vi "Initialize Attributes.vi"(8 "error in (no error)":errorcluster, 10 "Attribute Data":variant, 11 "CS++DIM-Client in":refnum<class "CS++DIM-Client.lvclass">) -> (0 "error out":errorcluster, 2 "Found?":bool, 3 "CS++DIM-Client out":refnum<class "CS++DIM-Client.lvclass">)   [LabVIEW 2016, in "CS++DIM-Client.lvlib" / "CS++DIM-Client.lvclass"]
doc: "Initialize object attribute.\n\nUnique resources should be allocated elsewhere!"
uses:
  CS++DIM-Client.lvclass
  CS++DIM-Client.lvclass/CS++DIM-Client.ctl
  CSPP_Core/Actors/CS++GUIActor/CS++GUIActor.lvclass
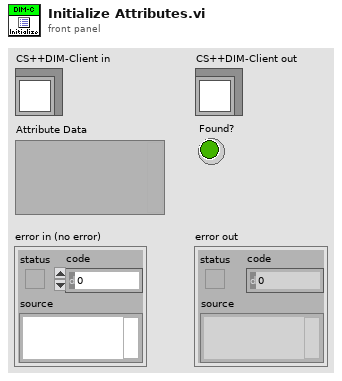
[diagram p1: front panel]
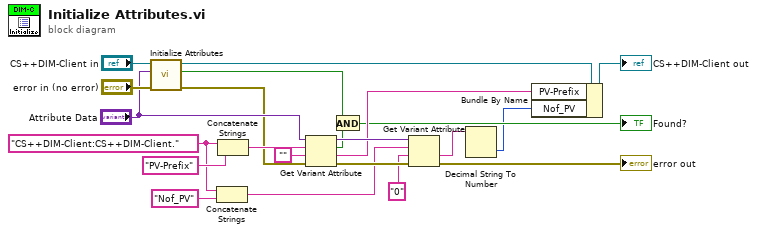
[diagram p0: block diagram]
diagram:
  w14 = "CS++DIM-Client:CS++DIM-Client."
  n1 = call-parent "Initialize Attributes.vi"("error in (no error)"="error in (no error)", "Attribute Data"="Attribute Data", "CS++GUIActor in"="CS++DIM-Client in") -> ("error out"=w10:errorcluster, "Found?"=w22:bool, "CS++GUIActor out"=w4:refnum<class "CS++DIM-Client.lvclass">)  [unwired: 6 in]
  n2 = Concatenate Strings(w14, "Nof_PV") -> (w12:string)
  n3 = Concatenate Strings(w14, "PV-Prefix") -> (w18:string)
  n4 = Get Variant Attribute(Variant="Attribute Data", name=w18, default value (empty Variant)="", error in=w10) -> (duplicate Variant=w16:variant, found=w6:bool, value=w8:string, error out=w15:errorcluster)
  n5 = And(x=w22, y=w6) -> (x .and. y?=→"Found?":bool)
  n6 = Get Variant Attribute(Variant=w16, name=w12, default value (empty Variant)="0", error in=w15) -> (value=w5:string, error out=→"error out":errorcluster)  [unwired: 2 out]
  n7 = Decimal String To Number(string=w5) -> (number=w1:i32)  [unwired: 2 in, 1 out]
  n8 = Bundle By Name(cluster=w4, "PV-Prefix"=w8, "Nof_PV"=w1) -> (→"CS++DIM-Client out":refnum<class "CS++DIM-Client.lvclass">)
